vi "ValidateOwner.vi"(8 "error in (no error)":errorcluster, 10 "Shared Key":string, 11 "SMO in":refnum<class "SMO.lvclass">) -> (0 "error out":errorcluster, 1 "not set":bool, 2 "key matched":bool, 3 "SMO out":refnum<class "SMO.lvclass">)   [LabVIEW 2021, in "smo.lvlib" / "SMO.lvclass"]
uses:
  SMO.lvclass
  SMO.lvclass/SMO.ctl
  Support/Attribute.Owner/Attribute.Owner.lvclass
  Support/Attribute.Owner/Attribute.Owner.lvclass/Attribute.Owner.ctl
  Support/Attribute.Owner/Read Shared Key.vi
  ReftoDVR--SMO.vi
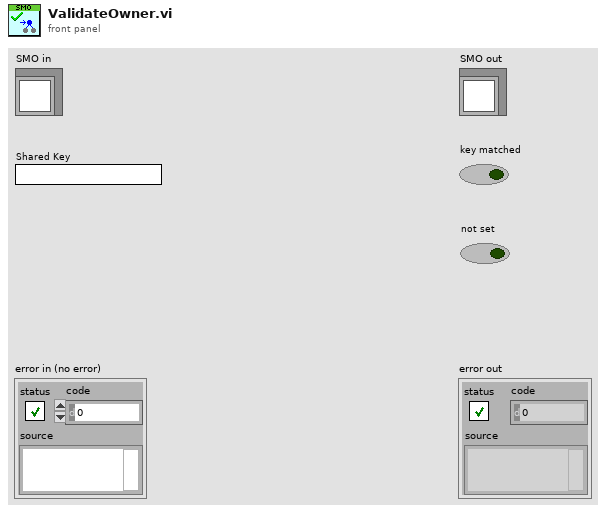
[diagram p1: front panel]
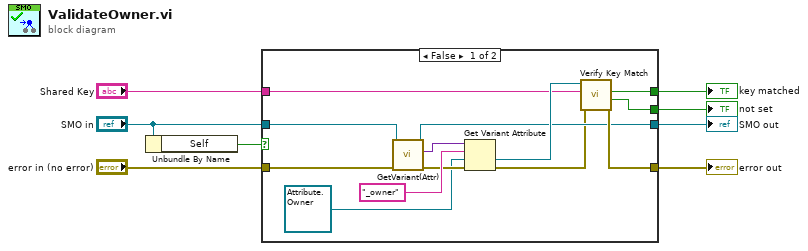
[diagram p0: block diagram]
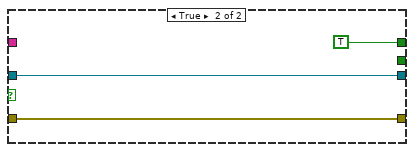
[diagram p2: hidden frame]
diagram:
  n1 = Unbundle By Name("SMO in") -> ("Self"=w2:bool)
  n2 = case shown="False" w2 {
    tunnel: "error in (no error)" -> [w13 w22]
    tunnel: [w10 w23] -> w7
    tunnel: "Shared Key" -> [w11 _]
    tunnel: [w21 w22] -> w5
    tunnel: [w20 TRUE ("key matched")] -> w4
    tunnel: "SMO in" -> [w14 w23]
    tunnel: [w19 _] -> w1
    frame False {
      n3 = call "GetVariant(Attr).vi"("error in (no error)"=w13, "SMO in"=w14) -> ("error out"=w16:errorcluster, "[Attributes]"=w18:variant, "SMO out"=w10:refnum<class "SMO.lvclass">)  [unwired: 7 in]
      n4 = Get Variant Attribute(Variant=w18, name="_owner", default value (empty Variant)=refnum<class "Attribute.Owner.lvclass"> refnum ("Attribute.Owner.lvclass"), error in=w16) -> (value=w12:refnum<class "Attribute.Owner.lvclass">, error out=w9:errorcluster)  [unwired: 2 out]
      n5 = call "Verify Key Match.vi"("error in (no error)"=w9, "Shared Key"=w11, "Attribute.Owner in"=w12) -> ("error out"=w21:errorcluster, "not set"=w19:bool, "key matched"=w20:bool)  [unwired: 5 in, 1 out]
    }
    frame True {
    }
  }
  "error out" <- w5
  "SMO out" <- w7
  "key matched" <- w4
  "not set" <- w1
